vi "ZCR filter zero.vi"(11 "waveform":waveform(dbl)) -> (3 "output waveform":waveform(dbl))   [LabVIEW 2020, in "Library Commun.lvlib" / "Nodon_ZCR.lvclass"]
uses:
  Nodon_ZCR.lvclass
  <vilib>/Analysis/baseanly.llb/Mean (DBL).vi
  Nodon_ZCR.lvclass/Nodon_ZCR.ctl
  <vilib>/Analysis/NI_AALBase.lvlib
panel:
  # "This VI filter the Zeros from the CH output of the SIN for ZCR measurement"
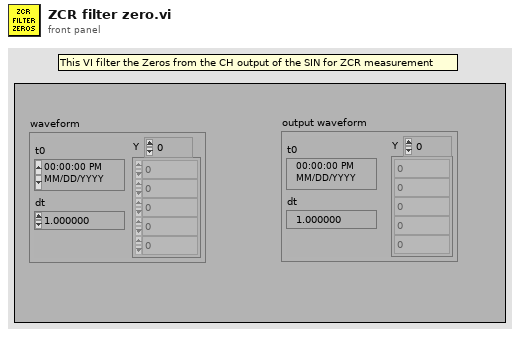
[diagram p1: front panel]
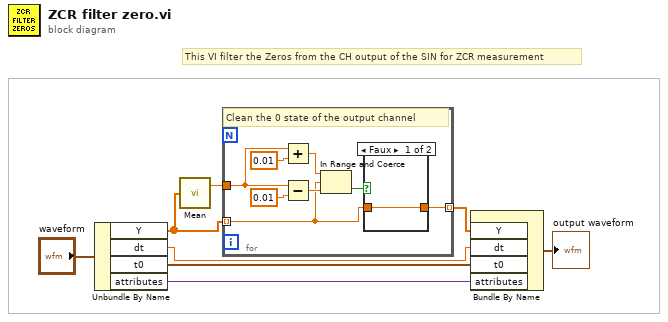
[diagram p0: block diagram]
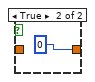
[diagram p2: hidden frame]
diagram:
  # "This VI filter the Zeros from the CH output of the SIN for ZCR measurement"
  n1 = Unbundle By Name("waveform") -> ("Y"=w3:dbl[], "dt"=w6:dbl, "t0"=w5:timestamp, "attributes"=w4:variant)
  n2 = call-poly <vilib>:"Mean.vi"("X"=w3) -> ("mean"=w8:dbl)  [unwired: 1 out]
  n3 = for {
    tunnel: w8 -> [w12]
    tunnel: [w10] -> w7 mode=indexing
    tunnel: w3 -> [w9] mode=indexing
    # "Clean the 0 state of the output channel"
    n4 = Add(x=w12, y=0.01) -> (x+y=w16:dbl)
    n5 = Subtract(x=w12, y=0.01) -> (x-y=w14:dbl)
    n6 = In Range and Coerce(upper limit=w16, x=w9, lower limit=w14) -> (In Range?=w11:bool)  [unwired: 1 out]
    n7 = case shown="Faux" w11 {
      tunnel: w9 -> [w17 _]
      tunnel: [w17 0] -> w10
      frame False {
      }
      frame True {
      }
    }
  }
  n8 = Bundle By Name("Y"=w7, "dt"=w6, "t0"=w5, "attributes"=w4) -> (→"output waveform":waveform(dbl))  [unwired: 1 in]
